vi "KINECT_Deadband.vi"(1 "Min":dbl, 2 "Max":dbl, 3 "Current Position":dbl, 4 "Deadband %":dbl) -> (0 "In Range?":bool)   [LabVIEW 2011]
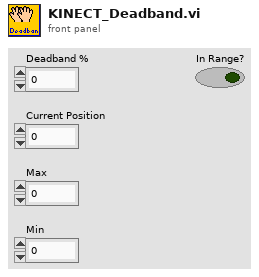
[diagram p1: front panel]
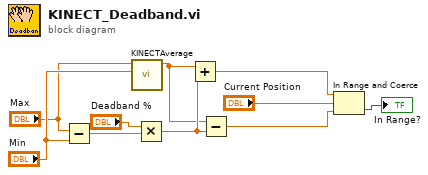
[diagram p0: block diagram]
diagram:
  n1 = Subtract(x="Max", y="Min") -> (x-y=w4:dbl)
  n2 = call "KINECTAverage.vi"("Min"="Min", "Max"="Max") -> ("Average"=w3:dbl)  [unwired: 8 in, 1 out]
  n3 = Multiply(x="Deadband %", y=w4) -> (x*y=w6:dbl)
  n4 = Add(x=w3, y=w6) -> (x+y=w1:dbl)
  n5 = Subtract(x=w3, y=w6) -> (x-y=w2:dbl)
  n6 = In Range and Coerce(upper limit=w1, x="Current Position", lower limit=w2) -> (In Range?=→"In Range?":bool)  [unwired: 1 out]
